vi "Check - In Project.vi"(11 "New QControl Info":refnum<data-value>) -> (0 "error out":errorcluster)   [LabVIEW 2015, in "New QControl Info.lvclass"]
doc: "<b> </b> <b> </b>\n©2016 Q Software Innovations, LLC (QSI)\nwritten by Quentin Alldredge\nproduced in LabVIEW 2015\n\nsupport@qsoftwareinnovations.com\nwww.qsoftwareinnovations.com\n\nAll rights reserved.\n\nRedistribution and use in source and binary forms, with or without modification, are permitted provided that the following conditions are met:\n\n * Redistributions of source code must retain the above copyright notice, this list of conditions and the following disclaimer.\n * Redistributions in binary form must reproduce the above copyright notice, this list of conditions and the following disclaimer in the documentation and/or other materials provided with the distribution.\n * Neither the name of Q Software Innovations, LLC. nor the names of its contributors may be used to endorse or promote products derived from this software without specific prior written permission.\n\nTHIS SOFTWARE IS PROVIDED BY THE COPYRIGHT HOLDERS AND CONTRIBUTORS \"AS IS\" AND ANY EXPRESS OR IMPLIED WARRANTIES, INCLUDING, BUT NOT LIMITED TO, THE IMPLIED WARRANTIES OF MERCHANTABILITY AND FITNESS FOR A PARTICULAR PURPOSE ARE DISCLAIMED. IN NO EVENT SHALL THE COPYRIGHT OWNER OR CONTRIBUTORS BE LIABLE FOR ANY DIRECT, INDIRECT, INCIDENTAL, SPECIAL, EXEMPLARY, OR CONSEQUENTIAL DAMAGES (INCLUDING, BUT NOT LIMITED TO, PROCUREMENT OF SUBSTITUTE GOODS OR SERVICES; LOSS OF USE, DATA, OR PROFITS; OR BUSINESS INTERRUPTION) HOWEVER CAUSED AND ON ANY THEORY OF LIABILITY, WHETHER IN CONTRACT, STRICT LIABILITY, OR TORT (INCLUDING NEGLIGENCE OR OTHERWISE) ARISING IN ANY WAY OUT OF THE USE OF THIS SOFTWARE, EVEN IF ADVISED OF THE POSSIBILITY OF SUCH DAMAGE."
uses:
  New QControl Info/New QControl Info.lvclass
  New QControl Info/New QControl Info.lvclass/New QControl Info.ctl
  New QControl Info/Read QControl Class Name.vi
  New QControl Info/Read Target Ref.vi
  New QControl Info/Read ProjectItem Ref.vi
  New QControl Info/Read Add to Location.vi
  <vilib>/ErrorRing/Error Ring.xnode
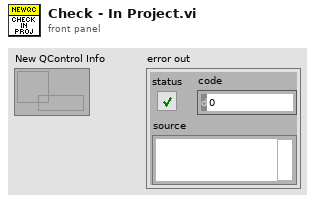
[diagram p1: front panel]
types:
  T1 = enum16{"Don't Add", "To Target", "To Project Item"}
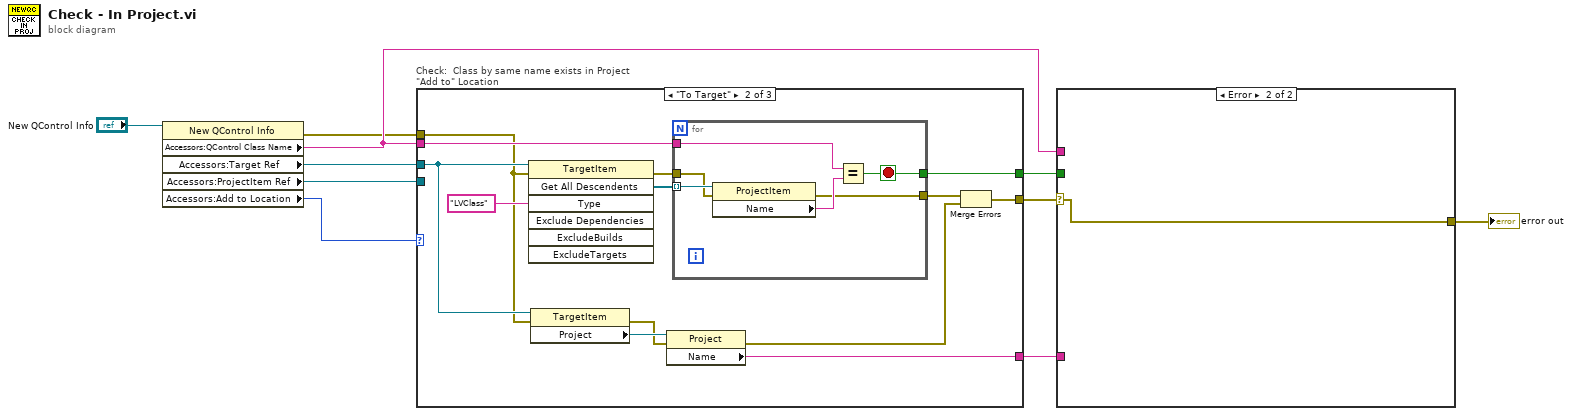
[diagram p0: block diagram]
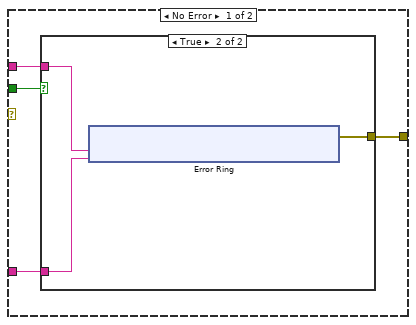
[diagram p2: hidden frame]
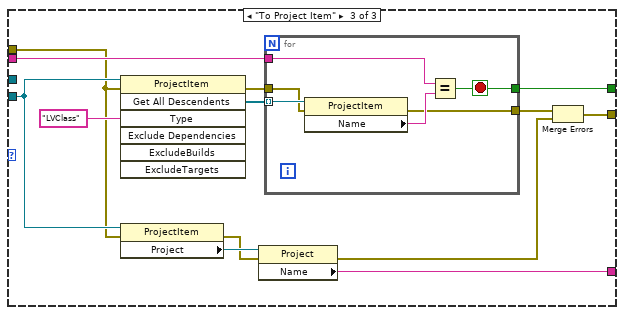
[diagram p5: hidden frame]
diagram:
  n1 = property class="New QControl Info"(reference="New QControl Info") -> (error out=w2:errorcluster, "Accessors:QControl Class Name"=w6:string, "Accessors:Target Ref"=w5:refnum<vi>, "Accessors:ProjectItem Ref"=w4:refnum<vi>, "Accessors:Add to Location"=w3:T1)  [unwired: 1 in, 1 out]
  n2 = case "Check:  Class by same name exists in Project \"Add to\" Location" shown="\"To Target\"" w3 {
    tunnel: w5 -> [_ w20 _]
    tunnel: w4 -> [_ _ w38]
    tunnel: w6 -> [_ w23 w42]
    tunnel: [_ w21 w40] -> w10
    tunnel: [_ w18 w37] -> w9
    tunnel: w2 -> [w11 w12 w33]
    tunnel: [w11 w15 w32] -> w1
    frame "Don't Add" {
    }
    frame "To Target" {
      n3 = invoke class="TargetItem" method="Get All Descendents"(reference=w20, error in=w12, "Type"="LVClass") -> (error out=w17:errorcluster, "All Descendents"=w22:refnum<vi>[])  [unwired: 4 in, 5 out]
      n4 = property class="TargetItem"(reference=w20, error in=w12) -> (error out=w14:errorcluster, "Project"=w19:refnum<vi>)  [unwired: 1 out]
      n5 = property class="Project"(reference=w19, error in=w14) -> (error out=w13:errorcluster, "Name"=w18:string)  [unwired: 1 out]
      n6 = for {
        tunnel: w23 -> [w29]
        tunnel: w22 -> [w30] mode=indexing
        tunnel: [w27] -> w21
        tunnel: w17 -> [w26]
        tunnel: [w25] -> w16
        stop <- w27 stop-if-true
        n7 = property class="ProjectItem"(reference=w30, error in=w26) -> (error out=w25:errorcluster, "Name"=w28:string)  [unwired: 1 out]
        n8 = Equal?(x=w29, y=w28) -> (x = y?=w27:bool)
      }
      n9 = Merge Errors(w16, w13) -> (w15:errorcluster)
    }
    frame "To Project Item" {
      n10 = invoke class="ProjectItem" method="Get All Descendents"(reference=w38, error in=w33, "Type"="LVClass") -> (error out=w36:errorcluster, "All Descendents"=w41:refnum<vi>[])  [unwired: 4 in, 5 out]
      n11 = property class="ProjectItem"(reference=w38, error in=w33) -> (error out=w34:errorcluster, "Project"=w39:refnum<vi>)  [unwired: 1 out]
      n12 = property class="Project"(reference=w39, error in=w34) -> (error out=w31:errorcluster, "Name"=w37:string)  [unwired: 1 out]
      n13 = for {
        tunnel: w42 -> [w48]
        tunnel: w41 -> [w49] mode=indexing
        tunnel: [w46] -> w40
        tunnel: w36 -> [w45]
        tunnel: [w44] -> w35
        stop <- w46 stop-if-true
        n14 = property class="ProjectItem"(reference=w49, error in=w45) -> (error out=w44:errorcluster, "Name"=w47:string)  [unwired: 1 out]
        n15 = Equal?(x=w48, y=w47) -> (x = y?=w46:bool)
      }
      n16 = Merge Errors(w35, w31) -> (w32:errorcluster)
    }
  }
  n17 = case shown="Error" w1 {
    selector: w1 -> [_ w63]
    tunnel: w10 -> [w53 _]
    tunnel: w9 -> [w52 _]
    tunnel: [w51 w63] -> w8
    tunnel: w6 -> [w50 _]
    frame No Error {
      n18 = case shown="True" w53 {
        tunnel: w52 -> [_ w56]
        tunnel: w50 -> [_ w55]
        tunnel: [_ w54] -> w51
        frame False {
        }
        frame True {
          n19 = xnode "Error Ring"("parameter 0"=w55, "parameter 1"=w56) -> ("error out"=w54:errorcluster)
        }
      }
    }
    frame Error {
    }
  }
  "error out" <- w8
